vi "Teleop.vi"(10 "Match Info":T1={"Autonomous Elapsed Seconds"=0.0, "TeleOp Elapsed Seconds"=0.0, "Disabled Elapsed Seconds"=0.0, "Visited Autonomous"=FALSE, "Visited TeleOp"=FALSE, "Visited Disabled"=FALSE, "Autonomous Settings"={"Autonomous Style"=enum."Independent", "VI Refnum"=refnum}}, 11 "Call Context":T2) -> ()   [LabVIEW 2016]
doc: "This VI is called for each TeleOp packet received from the DS where the robot is not disabled. It is often used to read from the joysticks and update I/O or to update setpoints for timed control loops. It should complete and return within 20 milliseconds or it may miss DS packets."
uses:
  <vilib>/Rock Robotics/WPI/DriverStation/WPI_DriverStationDerivedRobotMode.ctl
  <vilib>/Rock Robotics/WPI/DriverStation/WPI_DriverStationMatch Info.ctl
  <vilib>/Rock Robotics/WPI/Utilities/WPI_GetSetVariantRefNum.vi
  Robot Global Data.vi
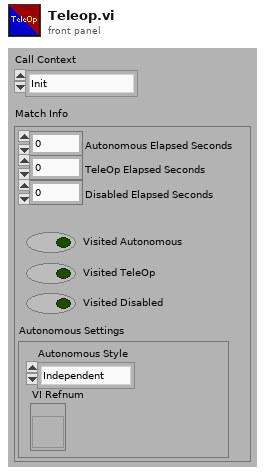
[diagram p1: front panel]
types:
  T1 = typedef "WPI_DriverStationMatch Info.ctl" = cluster{"Autonomous Elapsed Seconds":dbl, "TeleOp Elapsed Seconds":dbl, "Disabled Elapsed Seconds":dbl, "Visited Autonomous":bool, "Visited TeleOp":bool, "Visited Disabled":bool, "Autonomous Settings":cluster{"Autonomous Style":enum16{"Iterative", "Independent"}, "VI Refnum":refnum<vi>}}
  T2 = typedef "WPI_DriverStationDerivedRobotMode.ctl" = enum16{"Init", "Execute", "Stop"}
  T3 = cluster{"Top":bool, "Left":bool, "Right":bool, "Bottom":bool}
  T4 = typedef "WPI_JoystickDevRef.ctl" = cluster{"Device":T5}
  T5 = typedef "WPI_JoystickDeviceEnum.ctl" = enum16{"USB 0", "USB 1", "USB 2", "USB 3", "USB 4", "USB 5"}
  T6 = cluster{"Axes[0]":dbl, "Axes[1]":dbl, "Axes[2]":dbl, "Axes[3]":dbl, "Axes[4]":dbl, "Axes[5]":dbl, "Axes[6]":dbl, "Axes[7]":dbl, "Axes[8]":dbl}
  T7 = cluster{"Buttons[0]":bool, "Buttons[1]":bool, "Buttons[2]":bool, "Buttons[3]":bool, "Buttons[4]":bool, "Buttons[5]":bool, "Buttons[6]":bool, "Buttons[7]":bool, "Buttons[8]":bool}
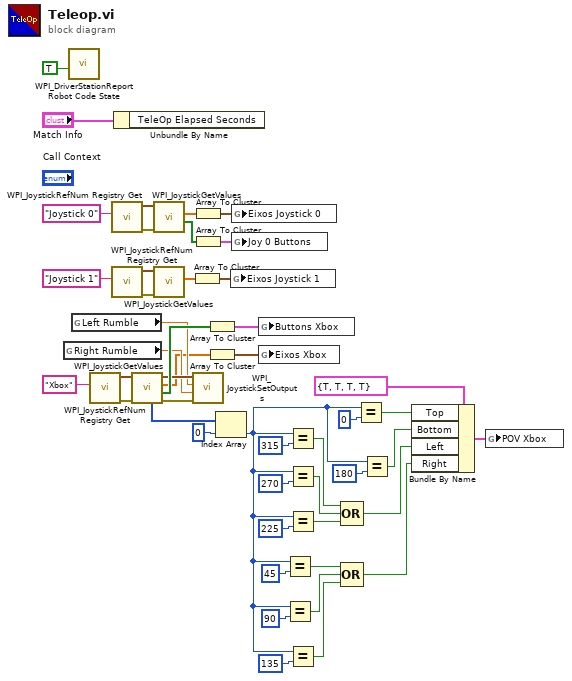
[diagram p0: block diagram]
diagram:
  n1 = global read "Robot Global Data.vi" "Right Rumble"() -> (w23:dbl)
  n2 = call <vilib>:"WPI_DriverStationReport Robot Code State.vi"("TeleOp"=TRUE ("Autonomous")) -> ()  [unwired: 10 in, 1 out]
  n3 = global read "Robot Global Data.vi" "Left Rumble"() -> (w22:dbl)
  n4 = call <vilib>:"WPI_JoystickRefNum Registry Get.vi"("refnum name"="Xbox") -> ("error out"=w35:errorcluster, "JoystickDevRef"=w36:T4)  [unwired: 9 in]
  n5 = call <vilib>:"WPI_JoystickRefNum Registry Get.vi"("refnum name"="Joystick 0") -> ("error out"=w45:errorcluster, "JoystickDevRef"=w46:T4)  [unwired: 9 in]
  n6 = call <vilib>:"WPI_JoystickRefNum Registry Get.vi"("refnum name"="Joystick 1") -> ("error out"=w41:errorcluster, "JoystickDevRef"=w42:T4)  [unwired: 9 in]
  n7 = Unbundle By Name("Match Info") -> ()  [unwired: 1 out]
  n8 = call <vilib>:"WPI_JoystickGetValues.vi"("error in (no error)"=w35, "JoystickDevRef"=w36) -> ("error out"=w24:errorcluster, "Buttons"=w33:bool[], "Axes"=w21:dbl[], "JoystickDevRef"=w25:T4, "POVs"=w31:i16[])  [unwired: 5 in]
  n9 = call <vilib>:"WPI_JoystickGetValues.vi"("error in (no error)"=w45, "JoystickDevRef"=w46) -> ("Buttons"=w4:bool[], "Axes"=w44:dbl[])  [unwired: 5 in, 3 out]
  n10 = call <vilib>:"WPI_JoystickGetValues.vi"("error in (no error)"=w41, "JoystickDevRef"=w42) -> ("Axes"=w40:dbl[])  [unwired: 5 in, 4 out]
  n11 = Array To Cluster(array=w40) -> (cluster=w39:T6)
  n12 = Array To Cluster(array=w44) -> (cluster=w43:T6)
  n13 = Array To Cluster(array=w4) -> (cluster=w3:T7)
  n14 = call <vilib>:"WPI_JoystickSetOutputs.vi"("error in (no error)"=w24, "Right Rumble"=w23, "Left Rumble"=w22, "JoystickDevRef"=w25) -> ()  [unwired: 6 in, 2 out]
  n15 = Array To Cluster(array=w33) -> (cluster=w32:T7)
  n16 = Array To Cluster(array=w21) -> (cluster=w20:T6)
  n17 = Index Array(array=w31, index=0) -> (element=w5:i16)
  n18 = global write "Robot Global Data.vi" "Eixos Joystick 1"(w39) -> ()
  n19 = global write "Robot Global Data.vi" "Eixos Joystick 0"(w43) -> ()
  n20 = global write "Robot Global Data.vi" "Joy 0 Buttons"(w3) -> ()
  n21 = global write "Robot Global Data.vi" "Buttons Xbox"(w32) -> ()
  n22 = global write "Robot Global Data.vi" "Eixos Xbox"(w20) -> ()
  n23 = Equal?(x=w5, y=i16 45) -> (x = y?=w17:bool)
  n24 = Equal?(x=w5, y=i16 90) -> (x = y?=w18:bool)
  n25 = Equal?(x=w5, y=i16 315) -> (x = y?=w11:bool)
  n26 = Equal?(x=w5, y=i16 270) -> (x = y?=w12:bool)
  n27 = Equal?(x=w5, y=i16 225) -> (x = y?=w13:bool)
  n28 = Equal?(x=w5, y=i16 135) -> (x = y?=w19:bool)
  n29 = Compound Arithmetic op=OR(w11, w12, w13) -> (w7:bool)
  n30 = Compound Arithmetic op=OR(w17, w18, w19) -> (w6:bool)
  n31 = Equal?(x=w5, y=i16 0) -> (x = y?=w2:bool)
  n32 = Equal?(x=w5, y=i16 180) -> (x = y?=w1:bool)
  n33 = Bundle By Name(cluster=T3 {"Top"=TRUE, "Left"=TRUE, "Right"=TRUE, "Bottom"=TRUE} ("input cluster"), "Top"=w2, "Bottom"=w1, "Left"=w7, "Right"=w6) -> (w26:T3)
  n34 = global write "Robot Global Data.vi" "POV Xbox"(w26) -> ()
